vi "OMV_WriteToUART.vi"(8 "error in":errorcluster, 9 "Text to write":string, 11 "VISA resource name":refnum<visa-resource-name>) -> (0 "error out":errorcluster, 3 "VISA Refnum out":refnum<visa-resource-name>)   [LabVIEW 2017]
panel:
  out "Num loops":i32
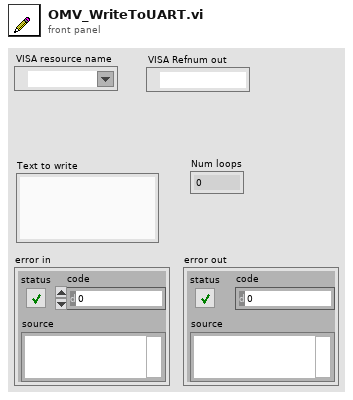
[diagram p1: front panel]
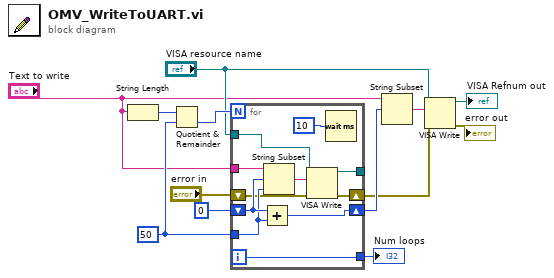
[diagram p0: block diagram]
diagram:
  w9 = 50 ("length (rest)")
  n1 = String Length(string="Text to write") -> (length=w8:i32)
  n2 = Quotient & Remainder(x=w8, y=w9) -> (floor(x/y)=w10:i32)  [unwired: 1 out]
  n3 = for {
    N: w10 -> [_]
    tunnel: "VISA resource name" -> [w24]
    tunnel: [w22] -> _
    tunnel: "Text to write" -> [w21]
    shift-right: [w18] -> w12
    shift-left: 0 -> [w19]
    tunnel: w9 -> [w17]
    tunnel: [w15] -> w6
    shift-right: [w23] -> w4
    shift-left: "error in" -> [w14]
    i -> [w15]
    n4 = Add(x=w19, y=w17) -> (x+y=w18:i32)
    n5 = String Subset(string=w21, offset (0)=w19, length (rest)=w17) -> (substring=w20:string)
    n6 = VISA Write(VISA resource name=w24, write buffer=w20, error in (no error)=w14) -> (VISA resource name out=w22:refnum<visa-resource-name>, error out=w23:errorcluster)  [unwired: 1 out]
    n7 = Wait (ms)(milliseconds to wait=u32 10) -> ()  [unwired: 1 out]
  }
  "Num loops" <- w6
  n8 = String Subset(string="Text to write", offset (0)=w12) -> (substring=w13:string)  [unwired: 1 in]
  n9 = VISA Write(VISA resource name="VISA resource name", write buffer=w13, error in (no error)=w4) -> (VISA resource name out=→"VISA Refnum out":refnum<visa-resource-name>, error out=→"error out":errorcluster)  [unwired: 1 out]
